vi "2D-array-to-cluster.vi"(1 "2D Array":dbl[][](array[numeric])) -> (0 "Cluster":T1)   [LabVIEW 2015]
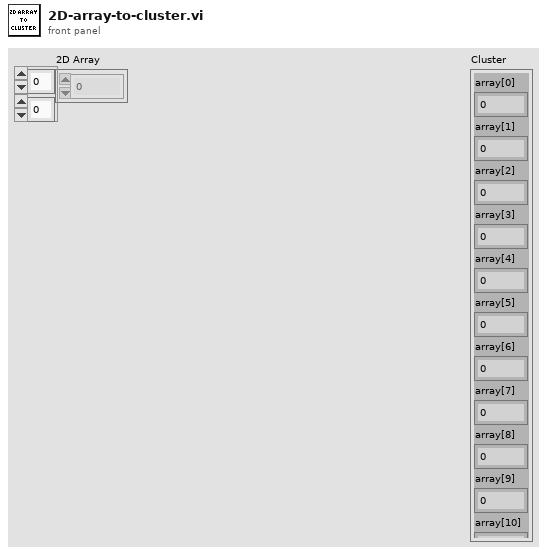
[diagram p1: front panel]
types:
  T1 = cluster{"array[0]":dbl, "array[1]":dbl, "array[2]":dbl, "array[3]":dbl, "array[4]":dbl, "array[5]":dbl, "array[6]":dbl, "array[7]":dbl, "array[8]":dbl, "array[9]":dbl, "array[10]":dbl, "array[11]":dbl, "array[12]":dbl, "array[13]":dbl, "array[14]":dbl, "array[15]":dbl, "array[16]":dbl, "array[17]":dbl, "array[18]":dbl, "array[19]":dbl, "array[20]":dbl, "array[21]":dbl, "array[22]":dbl, "array[23]":dbl, "array[24]":dbl, "array[25]":dbl, "array[26]":dbl, "array[27]":dbl, "array[28]":dbl, "array[29]":dbl, "array[30]":dbl, "array[31]":dbl}
  T2 = cluster{"2D Array[0]":dbl, "2D Array[1]":dbl, "2D Array[2]":dbl, "2D Array[3]":dbl, "2D Array[4]":dbl, "2D Array[5]":dbl, "2D Array[6]":dbl, "2D Array[7]":dbl, "2D Array[8]":dbl, "2D Array[9]":dbl, "2D Array[10]":dbl, "2D Array[11]":dbl, "2D Array[12]":dbl, "2D Array[13]":dbl, "2D Array[14]":dbl, "2D Array[15]":dbl, "2D Array[16]":dbl, "2D Array[17]":dbl, "2D Array[18]":dbl, "2D Array[19]":dbl, "2D Array[20]":dbl, "2D Array[21]":dbl, "2D Array[22]":dbl, "2D Array[23]":dbl, "2D Array[24]":dbl, "2D Array[25]":dbl, "2D Array[26]":dbl, "2D Array[27]":dbl, "2D Array[28]":dbl, "2D Array[29]":dbl, "2D Array[30]":dbl, "2D Array[31]":dbl}
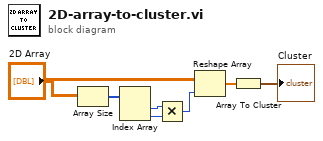
[diagram p0: block diagram]
diagram:
  n1 = Array Size(array="2D Array") -> (size(s)=w6:i32[])
  n2 = Index Array(array=w6) -> (element #1=w4:i32, element #2=w5:i32)  [unwired: 2 in]
  n3 = Multiply(x=w4, y=w5) -> (x*y=w3:i32)
  n4 = Reshape Array("2D Array", w3) -> (w7:dbl[])
  n5 = Array To Cluster(array=w7) -> (cluster=→"Cluster":T2)
